vi "Measurement.vi"(8 "error in (no error)":errorcluster, 9 "Grandeza":string, 10 "Multiplicador":dbl, 11 "289 in":refnum<class "289.lvclass">) -> (0 "error out":errorcluster, 2 "Measurement":dbl, 3 "289 out":refnum<class "289.lvclass">)   [LabVIEW 2015, in "289.lvclass"]
doc: "VI used to measure Value using the multimeter"
uses:
  289.lvclass
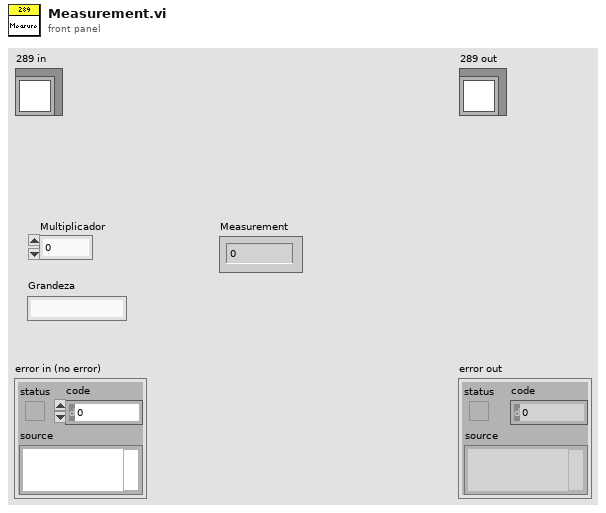
[diagram p1: front panel]
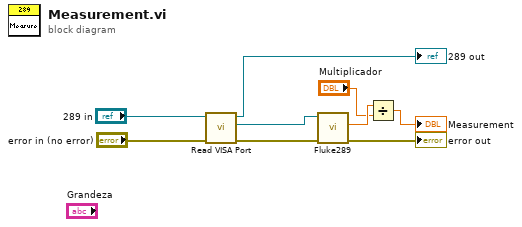
[diagram p0: block diagram]
diagram:
  n1 = call-dynamic "Read VISA Port.vi"("error in (no error)"="error in (no error)", "Device in"="289 in") -> ("error out"=w6:errorcluster, "VISA Port"=w4:refnum<visa-resource-name>, "Device out"=→"289 out":refnum<class "289.lvclass">)  [unwired: 7 in]
  n2 = call "Fluke289.vi"("error in (no error)"=w6, "VISA resource name"=w4) -> ("error out"=→"error out":errorcluster, "Measurement"=w3:dbl)  [unwired: 7 in, 1 out]
  n3 = Divide(x=w3, y="Multiplicador") -> (x/y=→"Measurement":dbl)
